vi "test_timeout 0 condition.vi"(8 "error in (no error)":errorcluster, 11 "TestCase in":refnum<class "Return Response Triggers.lvclass">) -> (0 "error out":errorcluster, 3 "TestCase out":refnum<class "Return Response Triggers.lvclass">)   [LabVIEW 2017, in "Return Response Triggers.lvclass"]
uses:
  Return Response Triggers.lvclass
  Libraries/SSH/Return Request Configuration.ctl
  Libraries/SSH/Response Configuration.ctl
  fb912344-4e5e-41e8-af55-9ce47520e721.vi
  <vilib>/addons/_JKI Toolkits/VI Tester/TestCase.llb/TestCase.lvclass
  Libraries/SSH/SSH.lvlib
  C:/Program Files (x86)/National Instruments/LabVIEW 2017/vi.lib/addons/_JKI Toolkits/VI Tester/TestCase.llb/TestCase.lvclass
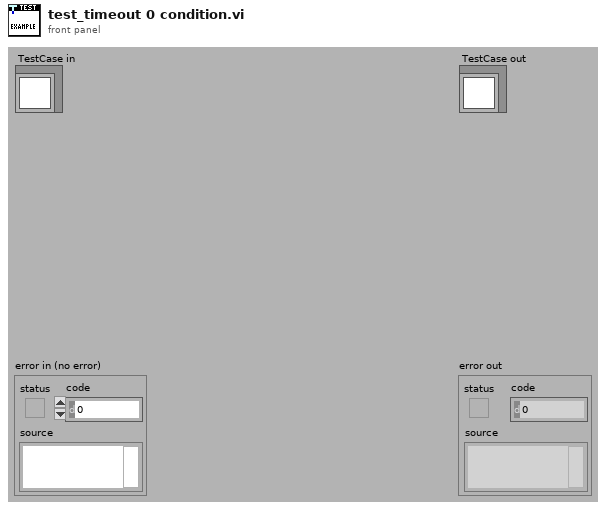
[diagram p1: front panel]
types:
  T1 = typedef "SSH.lvlib/Return Request Configuration.ctl" = cluster{"Response Configuration":T2, "Return Notifier":refnum<notifier>, "Response Requested":bool, "Command":string, "Initial Timer Value":u32}
  T2 = typedef "SSH.lvlib/Response Configuration.ctl" = cluster{"Expected Response":string, "Character Count Limit":i32, "Timeout (ms)":u32, "Update Response Config":bool}
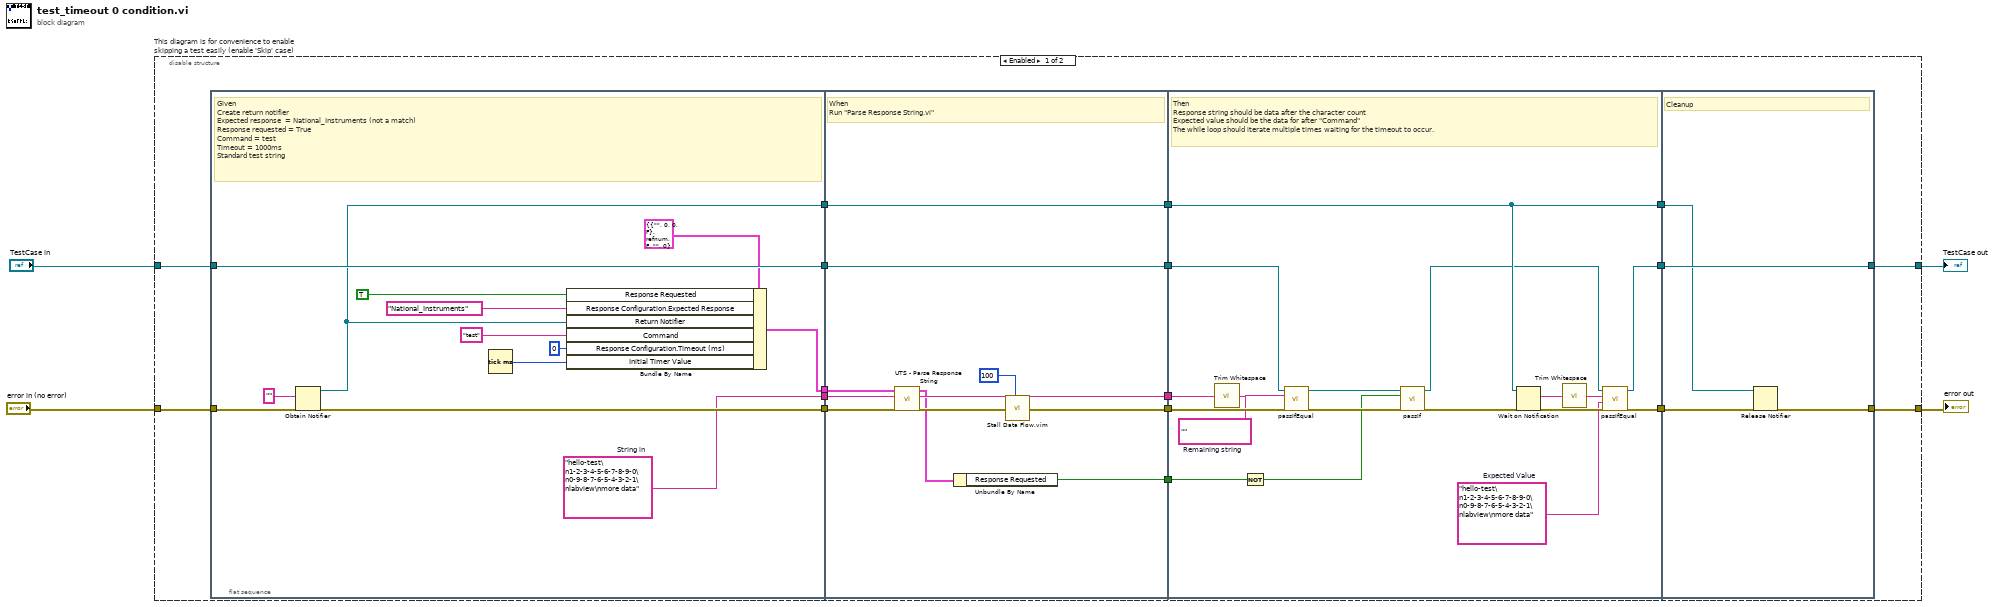
[diagram p0: block diagram]
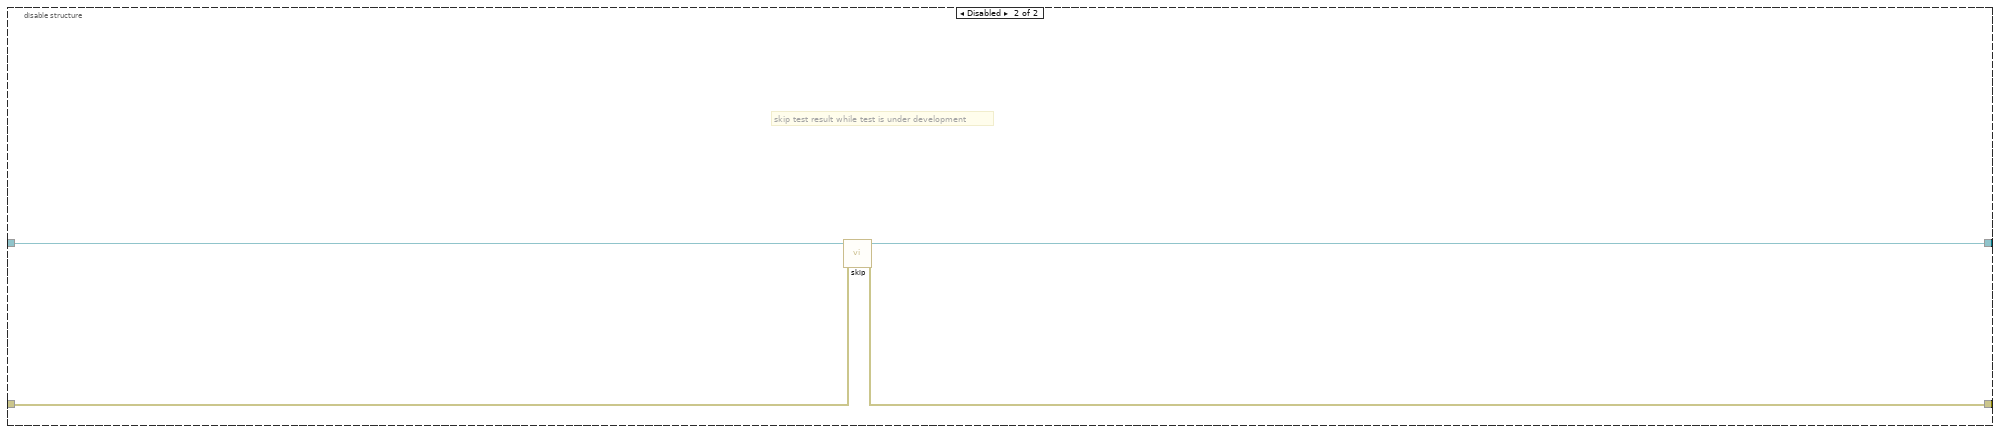
[diagram p2: hidden frame]
diagram:
  n1 = disable-structure "This diagram is for convenience to enable skipping a test easily (enable 'Skip' case)" shown="Enabled" {
    disable-tunnel: "TestCase in" -> [w14 w71]
    disable-tunnel: [w13 w69] -> w1
    disable-tunnel: [w12 w70] -> w3
    disable-tunnel: "error in (no error)" -> [w15 w68]
    frame Enabled {
      n2 = flat-sequence {
        tunnel: w15 -> [w31]
        tunnel: w14 -> [w34]
        tunnel: [w34] -> w21
        tunnel: [w30] -> w20
        tunnel: [w29] -> w11
        tunnel: [w25] -> w10
        tunnel: [w24] -> w9
        tunnel: [w45] -> w19
        tunnel: [w43] -> w18
        tunnel: w21 -> [w45]
        tunnel: w20 -> [w44]
        tunnel: w11 -> [w42]
        tunnel: w10 -> [w39]
        tunnel: w9 -> [w41]
        tunnel: [w40] -> w8
        tunnel: [w39] -> w7
        tunnel: [w35] -> w5
        tunnel: [w57] -> w17
        tunnel: [w58] -> w16
        tunnel: w19 -> [w63]
        tunnel: w18 -> [w62]
        tunnel: w8 -> [w60]
        tunnel: w7 -> [w54]
        tunnel: [w54] -> w6
        tunnel: w5 -> [w47]
        tunnel: [w65] -> w12
        tunnel: [w67] -> w13
        tunnel: w17 -> [w67]
        tunnel: w16 -> [w66]
        tunnel: w6 -> [w64]
        frame #0 {
          w24 = "hello-test\n1-2-3-4-5-6-7-8-9-0\n0-9-8-7-6-5-4-3-2-1\nlabview\nmore data"  # String in
          # "Given\nCreate return notifier\nExpected response  = National_Instruments (not a match)\nResponse requested = True\nCommand = test\nTimeout = 1000ms\nStandard test string"
          n3 = Obtain Notifier(notification data type="", error in (no error)=w31) -> (notifier out=w25:refnum<notifier>, error out=w30:errorcluster)  [unwired: 2 in, 1 out]
          n4 = Tick Count (ms)() -> (millisecond timer value=w22:u32)
          n5 = Bundle By Name(cluster=T1 {"Response Configuration"={"Expected Response"="", "Character Count Limit"=0, "Timeout (ms)"=0, "Update Response Config"=FALSE}, "Return Notifier"=refnum, "Response Requested"=FALSE, "Command"="", "Initial Timer Value"=0} ("Return Request in"), "Response Requested"=TRUE, "Response Configuration.Expected Response"="National_Instruments", "Return Notifier"=w25, "Command"="test", "Response Configuration.Timeout (ms)"=u32 0, "Initial Timer Value"=w22) -> (w29:T1)
        }
        frame #1 {
          # "When\nRun \"Parse Response String.vi\""
          n6 = call "UTS - Parse Response String.vi"("error in (no error)"=w44, "Response String in"=w41, "Return Request in"=w42) -> ("error out"=w38:errorcluster, "Response String out"=w40:string, "Return Request out"=w37:T1)  [unwired: 6 in]
          n7 = Unbundle By Name(w37) -> ("Response Requested"=w35:bool)
          n8 = call "Stall Data Flow.vim"("value in"=w38, "milliseconds to wait"=u32 100) -> ("value out"=w43:errorcluster)  [unwired: 1 out]
        }
        frame #2 {
          w53 = ""  # Remaining string
          w56 = "hello-test\n1-2-3-4-5-6-7-8-9-0\n0-9-8-7-6-5-4-3-2-1\nlabview\nmore data"  # Expected Value
          # "Then\nResponse string should be data after the character count\nExpected value should be the data for after \"Command\"\nThe while loop should iterate multiple times waiting for the timeout to occur."
          n9 = call <vilib>:"Trim Whitespace.vi"("string"=w60) -> ("trimmed string"=w52:string)  [unwired: 1 in]
          n10 = Not(x=w47) -> (.not. x?=w46:bool)
          n11 = call-dynamic "passIfEqual.vi"("error in (no error)"=w62, "y"=w53, "x"=w52, "TestCase in"=w63) -> ("error out"=w61:errorcluster, "TestCase out"=w49:refnum<class "Return Response Triggers.lvclass">)  [unwired: 6 in]
          n12 = call-dynamic "passIf.vi"("error in (no error)"=w61, "pass"=w46, "TestCase in"=w49) -> ("error out"=w50:errorcluster, "TestCase out"=w48:refnum<class "Return Response Triggers.lvclass">)  [unwired: 7 in]
          n13 = Wait on Notification(notifier=w54, error in (no error)=w50) -> (notification=w55:string, error out=w59:errorcluster)  [unwired: 2 in, 2 out]
          n14 = call <vilib>:"Trim Whitespace.vi"("string"=w55) -> ("trimmed string"=w51:string)  [unwired: 1 in]
          n15 = call-dynamic "passIfEqual.vi"("error in (no error)"=w59, "y"=w56, "x"=w51, "TestCase in"=w48) -> ("error out"=w58:errorcluster, "TestCase out"=w57:refnum<class "Return Response Triggers.lvclass">)  [unwired: 6 in]
        }
        frame #3 {
          # "Cleanup"
          n16 = Release Notifier(notifier=w64, error in (no error)=w66) -> (error out=w65:errorcluster)  [unwired: 1 in, 2 out]
        }
      }
    }
    frame Disabled {
      # "skip test result while test is under development"
      n17 = call <vilib>:"skip.vi"("error in (no error)"=w68, "TestCase in"=w71) -> ("error out"=w70:errorcluster, "TestCase out"=w69:refnum<class "Return Response Triggers.lvclass">)  [unwired: 8 in]
    }
  }
  "error out" <- w3
  "TestCase out" <- w1
